vi "lab 2.1.vi"() -> ()   [LabVIEW 2020]
panel:
  in  "Numeric":dbl
  out "Waveform Graph":dynamicdata(graph)
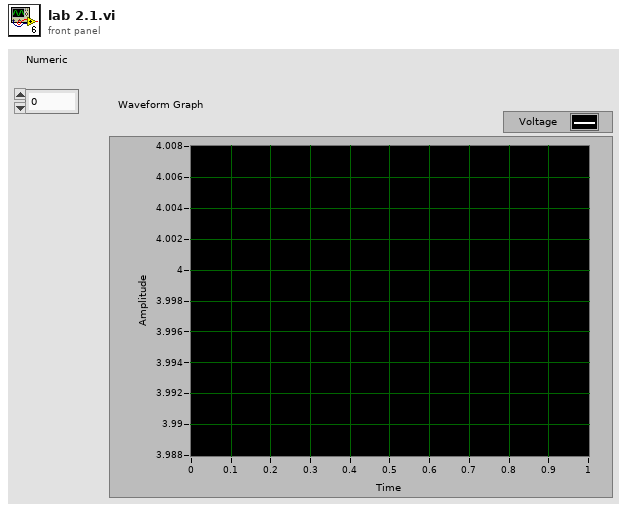
[diagram p1: front panel]
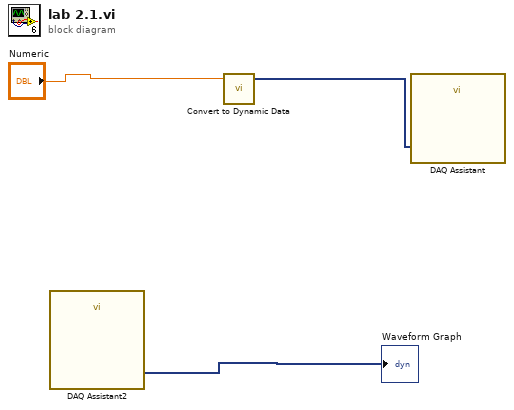
[diagram p0: block diagram]
diagram:
  n1 = call "DAQ Assistant2"() -> ("data"=→"Waveform Graph":dynamicdata)  [unwired: 17 in, 2 out]
  n2 = call "Convert to Dynamic Data"("Double"="Numeric") -> ("Dynamic Data Type"=w3:dynamicdata)  [unwired: 3 in]
  n3 = call "DAQ Assistant"("data"=w3) -> ()  [unwired: 17 in, 2 out]
